vi "Restarts Sandbox New.vi"() -> ()   [LabVIEW 2013]
uses:
  Type Defs/CAN Mode.ctl
  Type Defs/Controller Names.ctl
  Type Defs/Controller List.ctl
  <vilib>/FPGAPlugInAG/sbRIO-9626/niLvFpga_Open_sbRIO-9626.vi
  <vilib>/rvi/interface/common/dynamic/niFpgaDynamicAddResources.vi
  <vilib>/rvi/interface/common/niFpgaWaitOnOcc.vi
  <vilib>/Utility/error.llb/Error Cluster From Error Code.vi
  <vilib>/rvi/errors/niLvFpgaAdjustHostInterfaceError.vi
  <vilib>/FPGAPlugInAG/Dynamic/niLvFpga_Reset_Dynamic.vi
  <vilib>/FPGAPlugInAG/Dynamic/niLvFpga_Run_Dynamic.vi
  <vilib>/rvi/interface/nirviOpenFPGA/nirviOpenFPGA.xnode
  FPGA/bitfiles/New Restarts Sandbox.lvbitx
  <vilib>/rvi/interface/nirviMethod/nirviMethod.xnode
  <vilib>/rvi/interface/nirviReadWriteControl/nirviReadWriteControl.xnode
  NiFpgaLv.dll
  <vilib>/rvi/interface/Simulation/niFpgaSimulationCallBeginRW.vi
  <vilib>/NI_Real-Time Target Support.lvlib
  <vilib>/FPGAPlugInAG/Dynamic/niLvFpga_ReadFifo_Dynamic.vi
  <vilib>/rvi/errors/niLvFpgaMergeErrorWithErrorCode.vi
  <vilib>/FPGAPlugInAG/Dynamic/niLvFpga_ConfigureFifo_Dynamic.vi
panel:
  out "RT rstrts":dbl
  out "FPGA rstrts":dbl
  in  "Tab Control":enum32{"Page 1", "Page 2"}(tab)
  out "Current Graph":dbl[](graph)
  out "Pressure Graph":dbl[](graph)
  out "Restarts Graph":dbl[](graph)
  out "graph":dbl[][](graph)
  out "Snapshot Graph":dbl[][](graph)
  in  "HighLimit":dbl=13614.0 format="%#_17g"
  in  "LowLimit":dbl=13208.0 format="%#_17g"
  in  "Trigger Span":i32=5
  out "Tracker":u32
  in  "Update Graphs":bool
  in  "Snapshot":bool
  out "Data Array":dbl[][](array[numeric])
  out "Pressure":dbl
  out "DetPres Starts":u32
  out "Current":fxp<+/-,28,17>
  out "Commanded Starts":i16
  in  "Position":i32=1
  in  "Seconds per Step":dbl=1.5 min=0.25 max=500.0 step=0.25
  out "Case":string
  out "Current Step":i32
  in  "Reset Restarts":bool
  in  "Profile":dbl[][](array[numeric])=[[1.25, 0.0, 0.0], [1.25, 650.0, 700.0]]
  in  "Run profile?":bool
  out "CFR 2":u64 format="%.0x"
  in  "Pressure":dbl min=0.0 max=800.0 step=1.0 format="%#_13g"
  out "CPU Usage:":dbl=7.74131899555212 format="%.1f"
  in  "CAN CMD":dbl min=0.0 max=800.0 step=1.0
  # "13238"
  # "13413"
  # "cmd"
  # "pres"
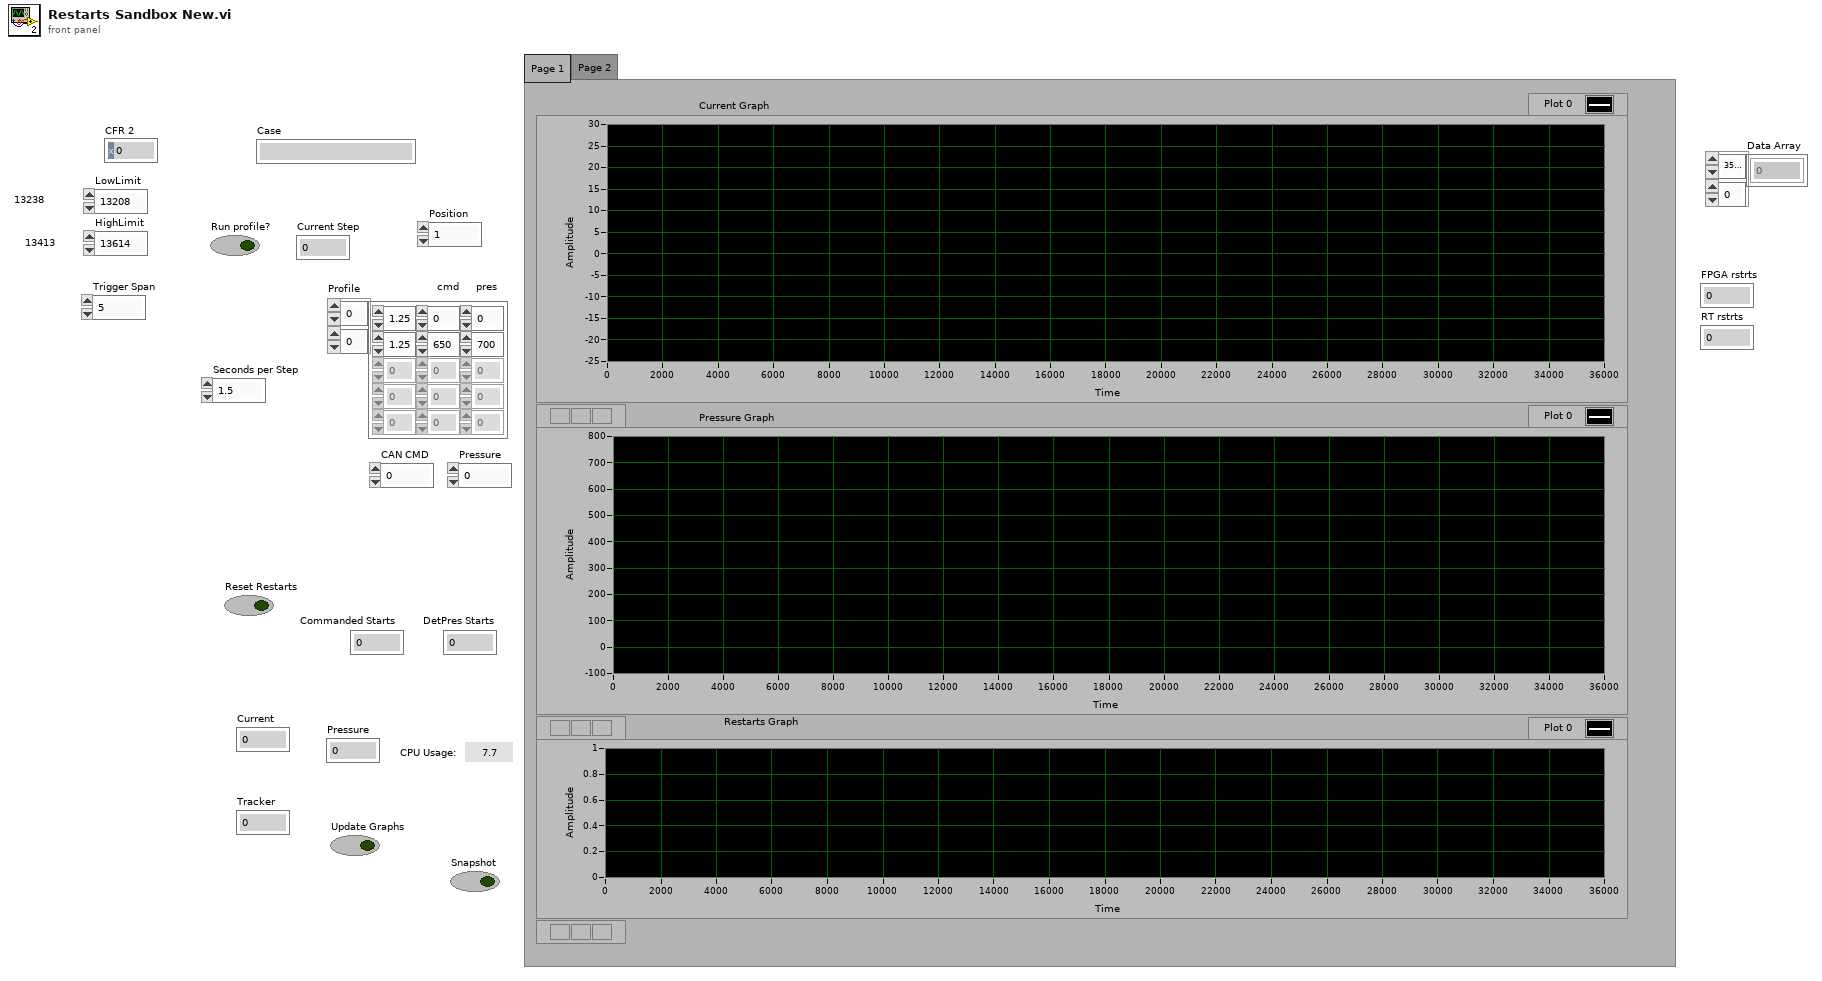
[diagram p1: front panel]
types:
  T1 = typedef "CAN Mode.ctl" = enum16{"Init", "Read", "Write", "Close"}
  T2 = cluster{"Container":dbl[], "Tracker":u32, "Curr1":dbl[], "Curr2":dbl[], "Curr3":dbl[], "Curr4":dbl[], "Curr5":dbl[], "Curr6":dbl[], "Pres1":dbl[], "Pres2":dbl[], "Pres3":dbl[], "Pres4":dbl[], "Pres5":dbl[], "Pres6":dbl[], "Restart1":dbl[], "Restart2":dbl[], "Restart3":dbl[], "Restart4":dbl[], "Restart5":dbl[], "Restart6":dbl[]}
  T3 = typedef "Controller Names.ctl" = enum16{"Kuhnke", "Conti", "Helbako", "TI PWM", "PSA", "Hella Gas", "Hella Diesel", "8 Comm", "10 Comm", "8 Comm Hella", "10 Comm Hella", "8 Comm Omron", "10 Comm Omron", "8 Comm Nissan", "10 Comm Nissan"}
  T4 = cluster{"Divide Value":u8, "Transfer Length (bits)":u8, "CS Asserted Polarity":bool, "Clock Polarity (CPOL)":bool, "Clock Phase (CPHA)":bool, "Lengthen MISO Setup":bool, "Direction Change Bit":u8, "MOSI Starts as Output":bool, "Tristatable MOSI":bool}
  T5 = typedef "Controller List.ctl" = cluster{"Controller Name":T3, "CommSeg":i32, "PWM?":bool, "Frequency":i32, "Low Command":dbl, "High Command":dbl, "Stop Command":dbl, "Command Step":dbl, "Solenoid Stop?":bool, "Controller?":bool}[]
  T6 = cluster{"Controller Name":T3, "CommSeg":i32, "PWM?":bool, "Frequency":i32, "Low Command":dbl, "High Command":dbl, "Stop Command":dbl, "Command Step":dbl, "Solenoid Stop?":bool, "Controller?":bool}
  T7 = typedef "NI_Real-Time Target Support.lvlib/RT CPU Load.ctl" = cluster{"Total (%)":dbl, "Time Critical (%)":dbl, "Timed Structures (%)":dbl, "High (%)":dbl, "Above Normal (%)":dbl, "Normal (%)":dbl, "Background (%)":dbl, "Idle (%)":dbl, "ISR (%)":dbl}
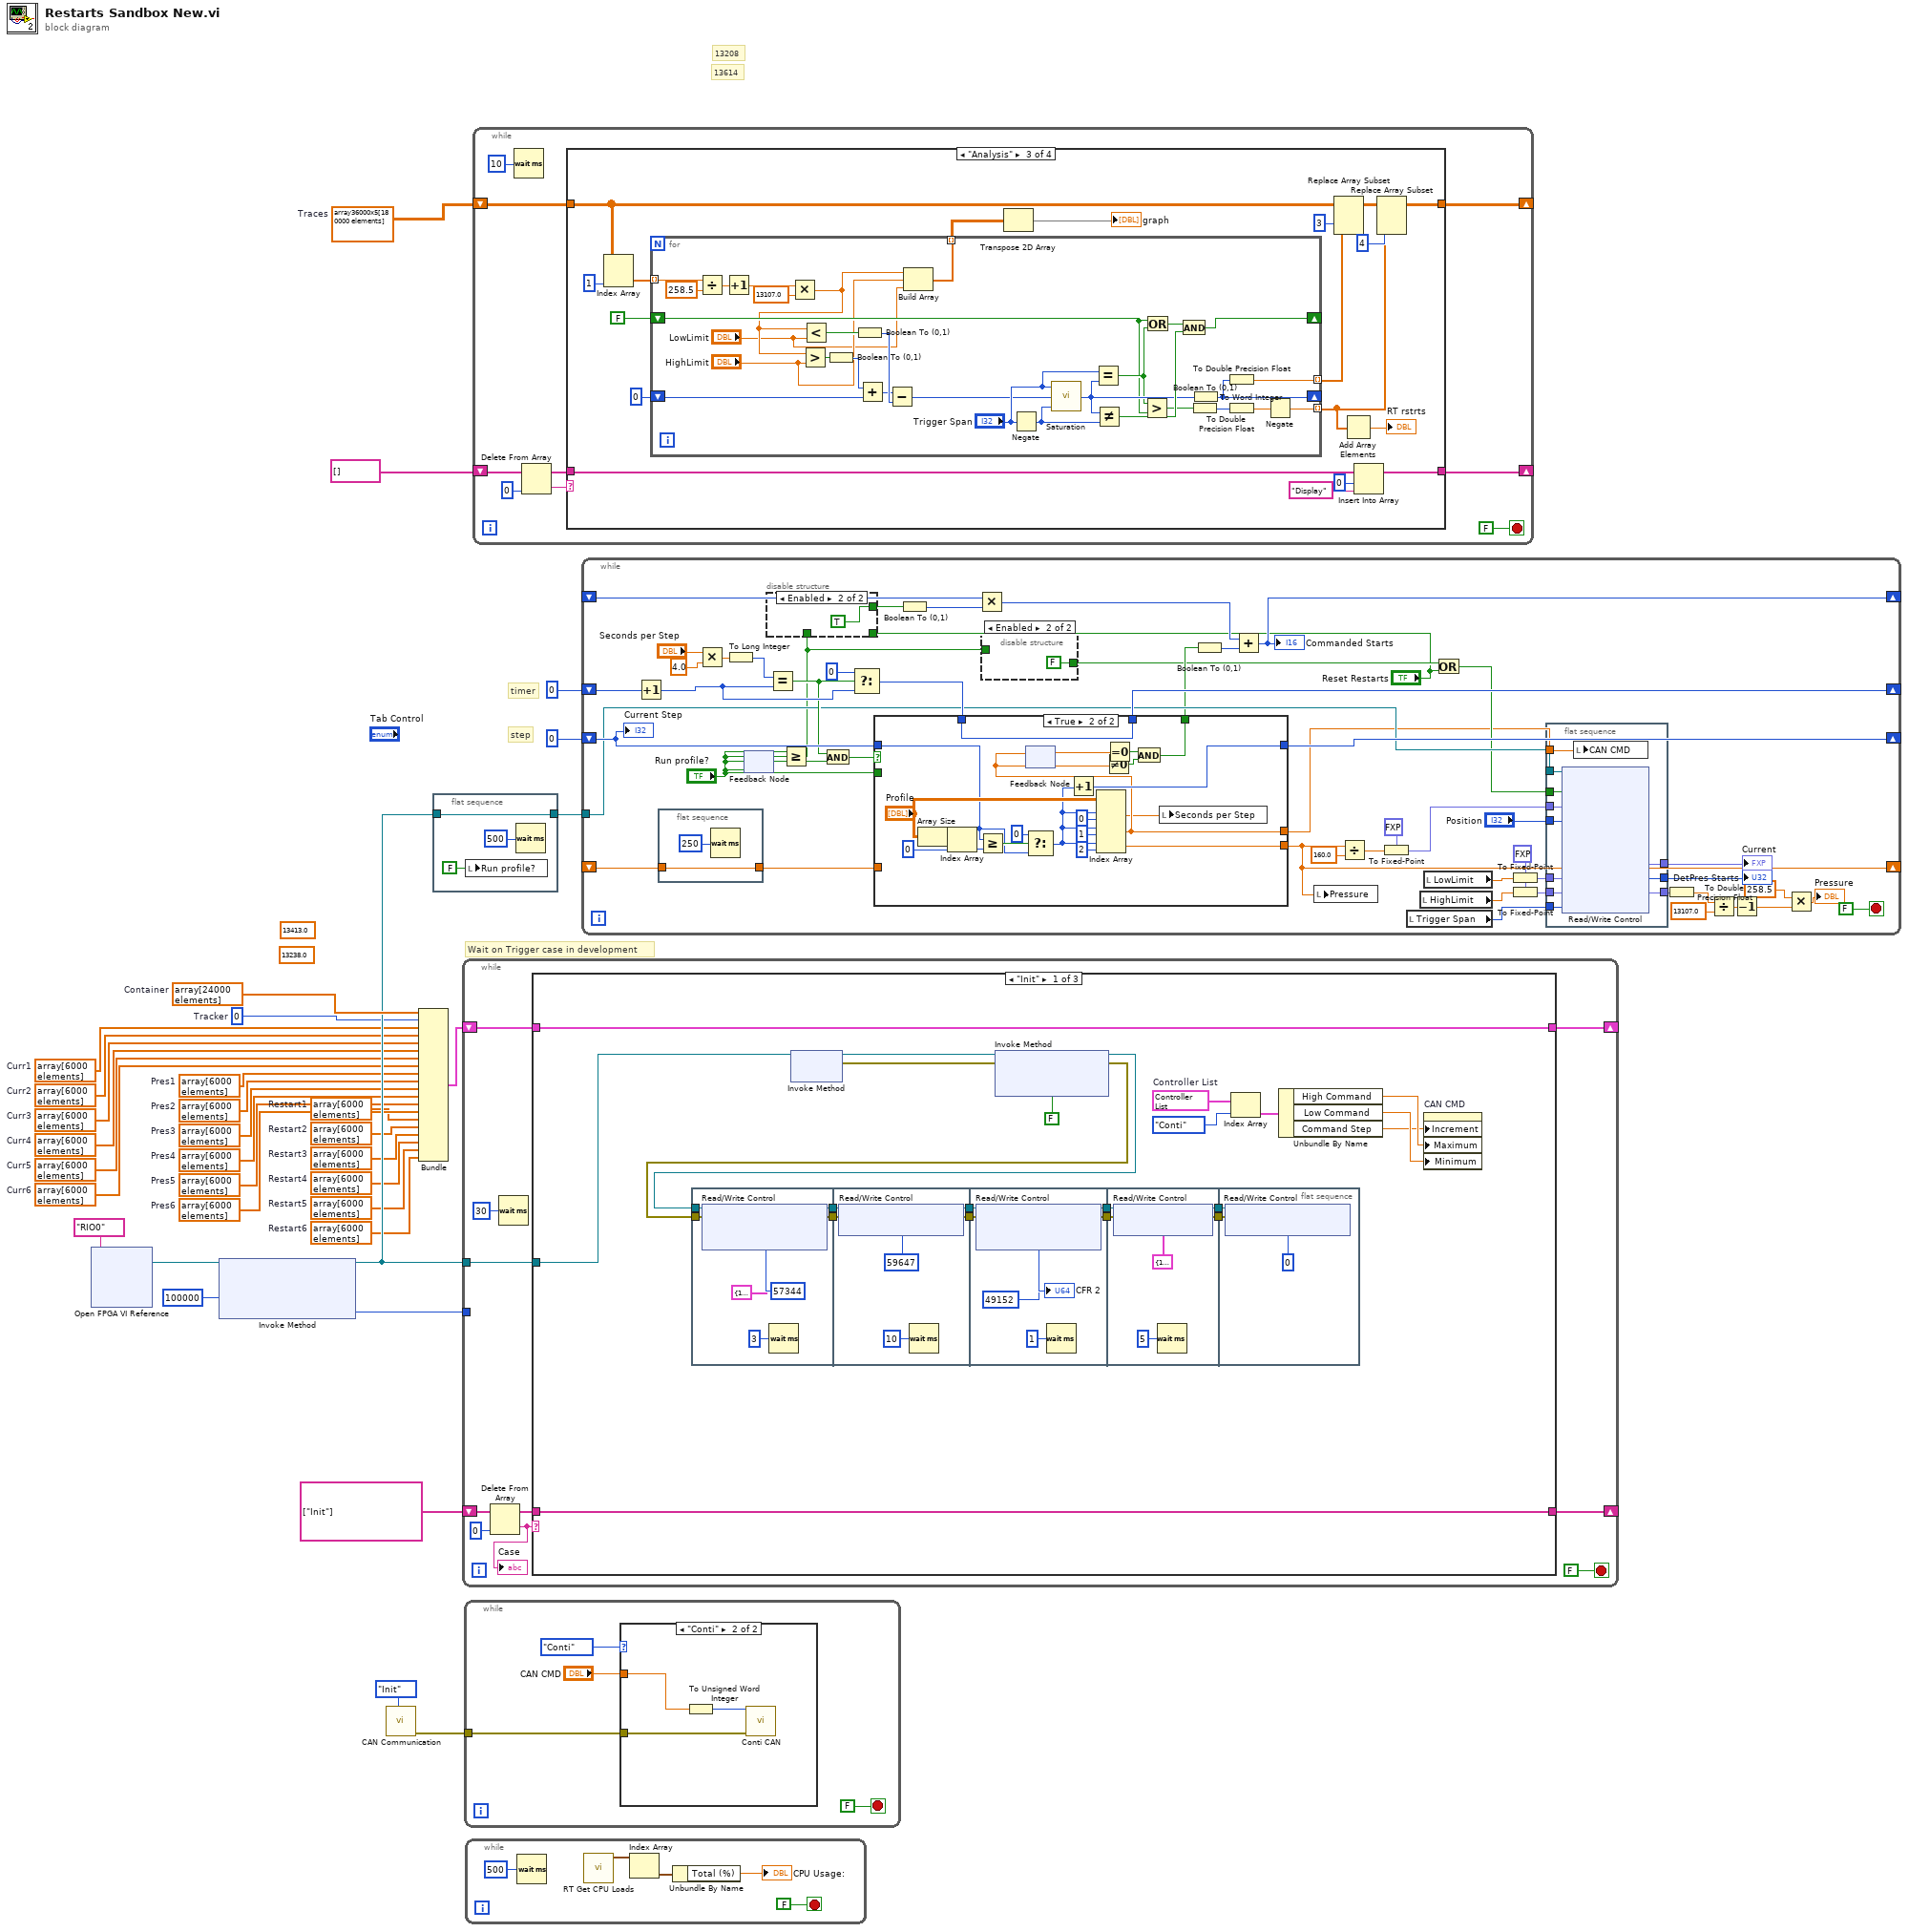
[diagram p0: block diagram]
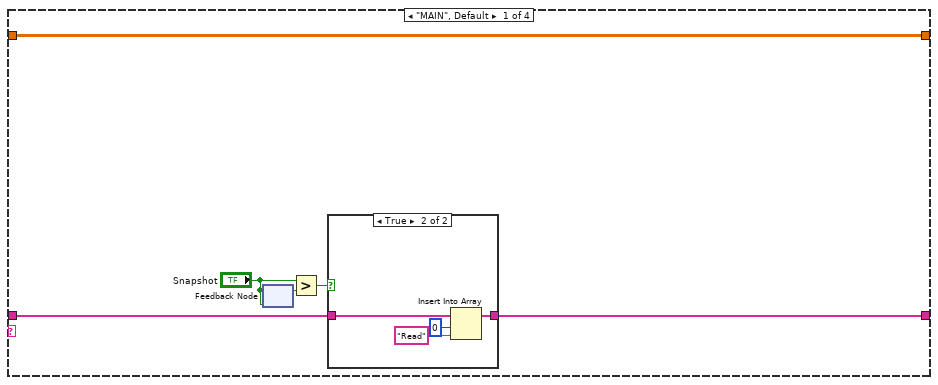
[diagram p2: hidden frame]
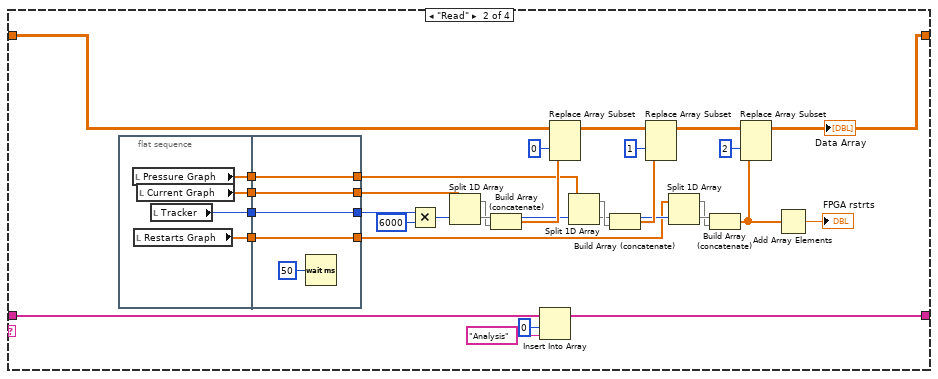
[diagram p4: hidden frame]
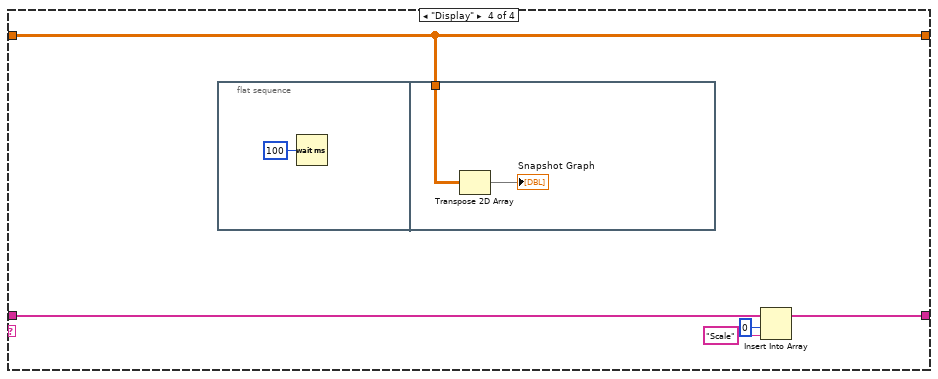
[diagram p5: hidden frame]
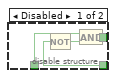
[diagram p6: hidden frame]
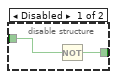
[diagram p7: hidden frame]
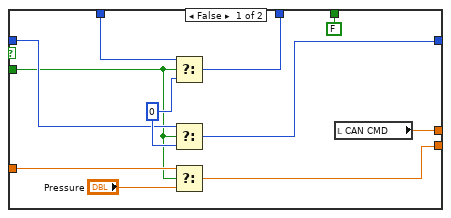
[diagram p8: hidden frame]
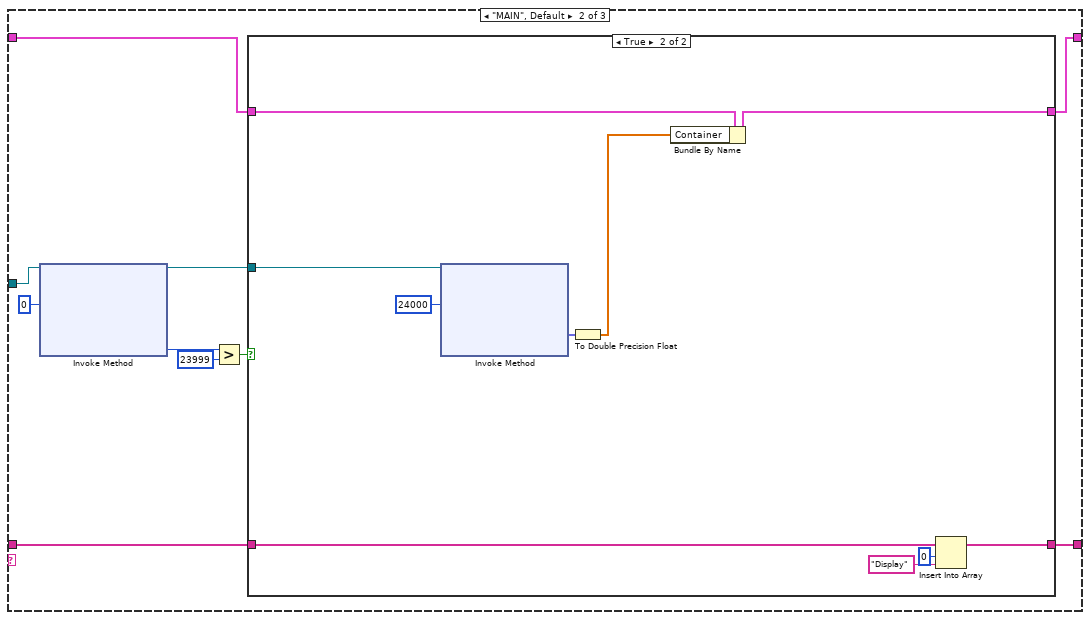
[diagram p9: hidden frame]
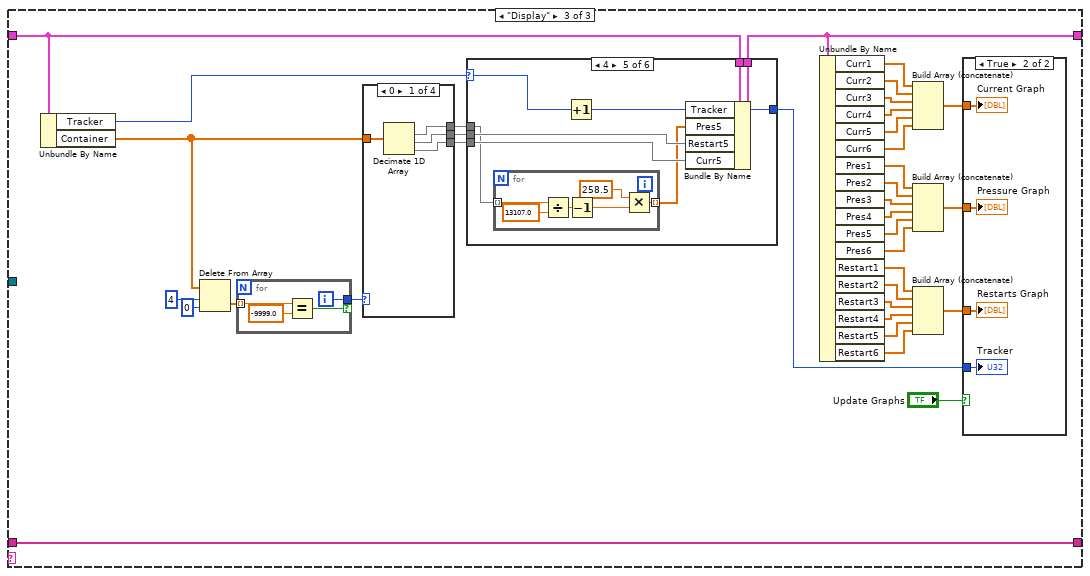
[diagram p11: hidden frame]
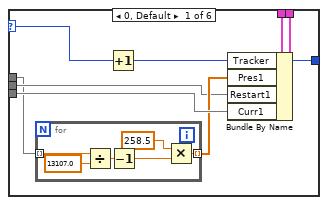
[diagram p13: hidden frame]
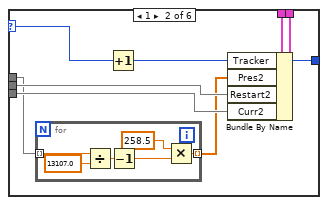
[diagram p14: hidden frame]
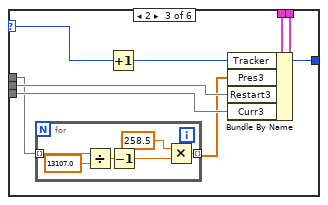
[diagram p15: hidden frame]
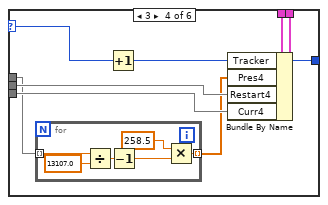
[diagram p16: hidden frame]
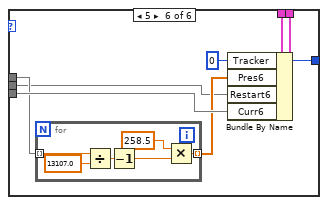
[diagram p17: hidden frame]
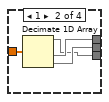
[diagram p18: hidden frame]
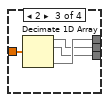
[diagram p19: hidden frame]
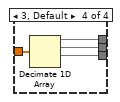
[diagram p20: hidden frame]
diagram:
  w2 = dbl[][] array36000x5[180000 elements]  # Traces
  w3 = dbl[] array[6000 elements]  # Restart6
  w4 = dbl[] array[6000 elements]  # Restart5
  w5 = dbl[] array[6000 elements]  # Restart4
  w6 = dbl[] array[6000 elements]  # Restart3
  w7 = dbl[] array[6000 elements]  # Restart2
  w8 = dbl[] array[6000 elements]  # Restart1
  w9 = dbl[] array[6000 elements]  # Pres6
  w10 = dbl[] array[6000 elements]  # Pres5
  w11 = dbl[] array[6000 elements]  # Pres4
  w12 = dbl[] array[6000 elements]  # Pres3
  w13 = dbl[] array[6000 elements]  # Pres2
  w14 = dbl[] array[6000 elements]  # Pres1
  w15 = dbl[] array[6000 elements]  # Curr6
  w16 = dbl[] array[6000 elements]  # Curr5
  w17 = dbl[] array[6000 elements]  # Curr4
  w18 = dbl[] array[6000 elements]  # Curr3
  w19 = dbl[] array[6000 elements]  # Curr2
  w20 = dbl[] array[6000 elements]  # Curr1
  (unwired) 13413.0 ("element")
  (unwired) 13238.0 ("element")
  w22 = u32 0  # Tracker
  w26 = dbl[] array[24000 elements]  # Container
  # "13614"
  # "13208"
  # "timer"
  # "step"
  # "Wait on Trigger case in development"
  n1 = xnode "Open FPGA VI Reference"("resource name"=tag "RIO0") -> ("FPGA VI Reference Out"=w28:refnum<k20>)  [unwired: 1 in, 1 out]
  n2 = xnode "Invoke Method"("FPGA VI Reference In"=w28, "Requested Depth"=u32 100000) -> ("FPGA VI Reference Out"=w25:refnum<k20>, "Actual Depth"=w27:u32)  [unwired: 1 in, 1 out]
  n3 = call "CAN Communication.vi"("CAN Mode"=CAN_Mode."Init") -> ("Error OUT"=w32:errorcluster)  [unwired: 10 in]
  n4 = Bundle("Container"=w26, "Tracker"=w22, "Curr1"=w20, "Curr2"=w19, "Curr3"=w18, "Curr4"=w17, "Curr5"=w16, "Curr6"=w15, "Pres1"=w14, "Pres2"=w13, "Pres3"=w12, "Pres4"=w11, "Pres5"=w10, "Pres6"=w9, "Restart1"=w8, "Restart2"=w7, "Restart3"=w6, "Restart4"=w5, "Restart5"=w4, "Restart6"=w3) -> (w30:T2)  [unwired: 1 in]
  n5 = flat-sequence {
    tunnel: w25 -> [w37]
    tunnel: [w37] -> w21
    frame #0 {
      n6 = local write "Run profile?"(FALSE ("Run profile?")) -> ()
      n7 = Wait (ms)(milliseconds to wait=u32 500) -> ()  [unwired: 1 out]
    }
  }
  n8 = while {
    shift-right: [w44] -> _
    shift-left: string[] ["Init"] -> [w47]
    shift-right: [w41] -> _
    shift-left: w30 -> [w42]
    tunnel: w25 -> [w40]
    tunnel: w27 -> [_]
    stop <- FALSE stop-if-true
    n9 = Delete From Array(array=w47, index=0) -> (deleted portion=w38:string, array with subset deleted=w45:string[])  [unwired: 1 in]
    "Case" <- w38
    n10 = Wait (ms)(milliseconds to wait=u32 30) -> ()  [unwired: 1 out]
    n11 = case shown="\"Init\"" w38 {
      tunnel: w45 -> [w69 w104 w154]
      tunnel: [w69 w103 w154] -> w44
      tunnel: w42 -> [w68 w101 w149]
      tunnel: [w68 w100 w121] -> w41
      tunnel: w40 -> [w67 w108 _]
      frame "Init" {
        w49 = T5 [{"Controller Name"=enum."Kuhnke", "CommSeg"=2, "PWM?"=TRUE, "Frequency"=100, "Low Command"=10.0, "High Command"=100.0, "Stop Command"=10.0, "Command Step"=0.1, "Solenoid Stop?"=FALSE, "Controller?"=FALSE}, {"Controller Name"=enum."Conti", "CommSeg"=2, "PWM?"=FALSE, "Frequency"=100, "Low Command"=0.0, "High Command"=800.0, "Stop Command"=0.0, "Command Step"=1.0, "Solenoid Stop?"=FALSE, "Controller?"=FALSE}, {"Controller Name"=enum."Helbako", "CommSeg"=2, "PWM?"=FALSE, "Frequency"=100, "Low Command"=0.0, "High Command"=100.0, "Stop Command"=0.0, "Command Step"=0.1, "Solenoid Stop?"=FALSE, "Controller?"=FALSE}, {"Controller Name"=enum."TI PWM", "CommSeg"=2, "PWM?"=TRUE, "Frequency"=100, "Low Command"=0.0, "High Command"=100.0, "Stop Command"=0.0, "Command Step"=0.1, "Solenoid Stop?"=FALSE, "Controller?"=FALSE}, {"Controller Name"=enum."PSA", "CommSeg"=2, "PWM?"=TRUE, "Frequency"=100, "Low Command"=5.0, "High Command"=95.0, "Stop Command"=5.0, "Command Step"=0.1, "Solenoid Stop?"=FALSE, "Controller?"=FALSE}, {"Controller Name"=enum."Hella Gas", "CommSeg"=2, "PWM?"=FALSE, "Frequency"=100, "Low Command"=0.0, "High Command"=800.0, "Stop Command"=0.0, "Command Step"=1.0, "Solenoid Stop?"=TRUE, "Controller?"=FALSE}, {"Controller Name"=enum."Hella Diesel", "CommSeg"=2, "PWM?"=FALSE, "Frequency"=100, "Low Command"=370.0, "High Command"=461.0, "Stop Command"=370.0, "Command Step"=1.0, "Solenoid Stop?"=TRUE, "Controller?"=FALSE}, {"Controller Name"=enum."8 Comm", "CommSeg"=8, "PWM?"=FALSE, "Frequency"=100, "Low Command"=0.0, "High Command"=1.0, "Stop Command"=0.0, "Command Step"=1.0, "Solenoid Stop?"=FALSE, "Controller?"=FALSE}, {"Controller Name"=enum."10 Comm", "CommSeg"=10, "PWM?"=FALSE, "Frequency"=100, "Low Command"=0.0, "High Command"=1.0, "Stop Command"=0.0, "Command Step"=1.0, "Solenoid Stop?"=FALSE, "Controller?"=FALSE}, {"Controller Name"=enum."8 Comm Hella", "CommSeg"=8, "PWM?"=TRUE, "Frequency"=150, "Low Command"=0.0, "High Command"=50.0, "Stop Command"=80.0, "Command Step"=0.1, "Solenoid Stop?"=FALSE, "Controller?"=FALSE}, {"Controller Name"=enum."10 Comm Hella", "CommSeg"=10, "PWM?"=TRUE, "Frequency"=150, "Low Command"=0.0, "High Command"=50.0, "Stop Command"=80.0, "Command Step"=0.1, "Solenoid Stop?"=FALSE, "Controller?"=FALSE}, {"Controller Name"=enum."8 Comm Omron", "CommSeg"=8, "PWM?"=TRUE, "Frequency"=150, "Low Command"=5.0, "High Command"=50.0, "Stop Command"=75.0, "Command Step"=0.1, "Solenoid Stop?"=FALSE, "Controller?"=FALSE}, {"Controller Name"=enum."10 Comm Omron", "CommSeg"=10, "PWM?"=TRUE, "Frequency"=150, "Low Command"=5.0, "High Command"=50.0, "Stop Command"=75.0, "Command Step"=0.1, "Solenoid Stop?"=FALSE, "Controller?"=FALSE}, {"Controller Name"=enum."8 Comm Nissan", "CommSeg"=8, "PWM?"=TRUE, "Frequency"=10, "Low Command"=50.0, "High Command"=90.0, "Stop Command"=50.0, "Command Step"=0.1, "Solenoid Stop?"=TRUE, "Controller?"=FALSE}, {"Controller Name"=enum."10 Comm Nissan", "CommSeg"=10, "PWM?"=TRUE, "Frequency"=10, "Low Command"=50.0, "High Command"=90.0, "Stop Command"=50.0, "Command Step"=0.1, "Solenoid Stop?"=TRUE, "Controller?"=FALSE}]  # Controller List
        n12 = flat-sequence {
          tunnel: w53 -> [w75]
          tunnel: w52 -> [w73]
          tunnel: [w76] -> w61
          tunnel: [w74] -> w60
          tunnel: w61 -> [w81]
          tunnel: w60 -> [w80]
          tunnel: [w79] -> w59
          tunnel: [w78] -> w58
          tunnel: w59 -> [w88]
          tunnel: w58 -> [w87]
          tunnel: [w86] -> w57
          tunnel: [w85] -> w56
          tunnel: w57 -> [w94]
          tunnel: w56 -> [w93]
          tunnel: [w91] -> w55
          tunnel: [w90] -> w54
          tunnel: w55 -> [w97]
          tunnel: w54 -> [w96]
          frame #0 {
            n13 = xnode "Read/Write Control"("FPGA VI Reference In"=w75, "error in"=w73, "AI16-23 Settings"=T4 {"Divide Value"=1, "Transfer Length (bits)"=16, "CS Asserted Polarity"=FALSE, "Clock Polarity (CPOL)"=TRUE, "Clock Phase (CPHA)"=FALSE, "Lengthen MISO Setup"=FALSE, "Direction Change Bit"=0, "MOSI Starts as Output"=FALSE, "Tristatable MOSI"=FALSE} ("Master Settings"), "AI16-23 Data to Write"=u64 57344 ("data to write")) -> ("FPGA VI Reference Out"=w76:refnum<k20>, "error out"=w74:errorcluster)
            n14 = Wait (ms)(milliseconds to wait=u32 3) -> ()  [unwired: 1 out]
          }
          frame #1 {
            n15 = xnode "Read/Write Control"("FPGA VI Reference In"=w81, "error in"=w80, "AI16-23 Data to Write"=u64 59647 ("data to write")) -> ("FPGA VI Reference Out"=w79:refnum<k20>, "error out"=w78:errorcluster)
            n16 = Wait (ms)(milliseconds to wait=u32 10) -> ()  [unwired: 1 out]
          }
          frame #2 {
            n17 = xnode "Read/Write Control"("FPGA VI Reference In"=w88, "error in"=w87, "AI16-23 Data to Write"=u64 49152 ("data to write")) -> ("FPGA VI Reference Out"=w86:refnum<k20>, "error out"=w85:errorcluster, "Read Data"=→"CFR 2":u64)
            n18 = Wait (ms)(milliseconds to wait=u32 1) -> ()  [unwired: 1 out]
          }
          frame #3 {
            n19 = xnode "Read/Write Control"("FPGA VI Reference In"=w94, "error in"=w93, "AI16-23 Settings"=T4 {"Divide Value"=1, "Transfer Length (bits)"=19, "CS Asserted Polarity"=FALSE, "Clock Polarity (CPOL)"=TRUE, "Clock Phase (CPHA)"=FALSE, "Lengthen MISO Setup"=FALSE, "Direction Change Bit"=0, "MOSI Starts as Output"=FALSE, "Tristatable MOSI"=FALSE} ("Master Settings")) -> ("FPGA VI Reference Out"=w91:refnum<k20>, "error out"=w90:errorcluster)
            n20 = Wait (ms)(milliseconds to wait=u32 5) -> ()  [unwired: 1 out]
          }
          frame #4 {
            n21 = xnode "Read/Write Control"("FPGA VI Reference In"=w97, "error in"=w96, "AI16-23 Data to Write"=u64 0) -> ()  [unwired: 2 out]
          }
        }
        n22 = xnode "Invoke Method"("FPGA VI Reference In"=w67) -> ("FPGA VI Reference Out"=w51:refnum<k20>, "error out"=w50:errorcluster)  [unwired: 1 in]
        n23 = xnode "Invoke Method"("FPGA VI Reference In"=w51, "error in"=w50, "Wait Until Done (F)"=FALSE) -> ("FPGA VI Reference Out"=w53:refnum<k20>, "error out"=w52:errorcluster)
        n24 = Index Array(array=w49, index=Controller_Names."Conti" ("Controller Type:")) -> (element=w63:T6)
        n25 = Unbundle By Name(w63) -> ("High Command"=w66:dbl, "Low Command"=w65:dbl, "Command Step"=w64:dbl)
        n26 = property on="CAN CMD" class="DigNum (strict)"("Increment"=w64, "Maximum"=w66, "Minimum"=w65) -> ()  [unwired: 2 in, 2 out]
      }
      frame "MAIN", Default {
        n27 = xnode "Invoke Method"("FPGA VI Reference In"=w108, "Number of Elements"=u32 0) -> ("FPGA VI Reference Out"=w99:refnum<k20>, "Elements Remaining"=w106:u32)  [unwired: 2 in, 2 out]
        n28 = Greater?(x=w106, y=u32 23999) -> (0:w102:bool)
        n29 = case shown="True" w102 {
          tunnel: w104 -> [w110 w118]
          tunnel: [w110 w117] -> w103
          tunnel: w101 -> [w109 w120]
          tunnel: [w109 w119] -> w100
          tunnel: w99 -> [_ w115]
          frame False {
          }
          frame True {
            n30 = xnode "Invoke Method"("FPGA VI Reference In"=w115, "Number of Elements"=u32 24000) -> ("Data"=w116:fxp<+/-,28,17>[])  [unwired: 2 in, 3 out]
            n31 = To Double Precision Float(number=w116) -> (double precision float=w113:dbl[])
            n32 = Bundle By Name(cluster=w120, "Container"=w113) -> (w119:T2)
            n33 = Insert Into Array(array=w118, index=0, new element="Display" ("new element/subarray")) -> (w117:string[])
          }
        }
      }
      frame "Display" {
        n34 = Unbundle By Name(w149) -> ("Tracker"=w124:u32, "Container"=w150:dbl[])
        n35 = Delete From Array(array=w150, length=4, index=0) -> (deleted portion=w152:dbl[])  [unwired: 1 out]
        n36 = for {
          tunnel: w152 -> [w261] mode=indexing
          tunnel: [w262] -> w151 if=w259
          i -> [w262]
          n37 = Equal?(x=w261, y=-9999.0) -> (x = y?=w259:bool)
        }
        n38 = case shown="0" w151 {
          tunnel: w150 -> [w246 w250 w254 w258]
          tunnel: [w245 w249 w253 w257] -> w127
          tunnel: [w244 w248 w252 w256] -> w126
          tunnel: [w243 w247 w251 w255] -> w125
          frame 0 {
            n39 = Decimate 1D Array(w246) -> (w245:dbl[], w244:dbl[], w243:dbl[])  [unwired: 1 out]
          }
          frame 1 {
            n40 = Decimate 1D Array(w250) -> (w247:dbl[], w249:dbl[], w248:dbl[])  [unwired: 1 out]
          }
          frame 2 {
            n41 = Decimate 1D Array(w254) -> (w252:dbl[], w251:dbl[], w253:dbl[])  [unwired: 1 out]
          }
          frame 3, Default {
            n42 = Decimate 1D Array(w258) -> (w257:dbl[], w256:dbl[], w255:dbl[])  [unwired: 1 out]
          }
        }
        n43 = case shown="4" w124 {
          selector: w124 -> [w164 w178 w192 w206 w220 _]
          tunnel: w127 -> [w161 w176 w189 w203 w217 w233]
          tunnel: w126 -> [w162 w177 w191 w205 w219 w231]
          tunnel: w125 -> [w166 w180 w194 w208 w222 w235]
          tunnel: w149 -> [w167 w181 w195 w209 w223 w236]
          tunnel: [w165 w179 w193 w207 w221 w234] -> w121
          tunnel: [w160 w174 w188 w202 w216 w230] -> w122
          frame 0, Default {
            n44 = for {
              tunnel: w161 -> [w169] mode=indexing
              tunnel: [w168] -> w163 mode=indexing
              n45 = Divide(x=w169, y=13107.0) -> (x/y=w171:dbl)
              n46 = Decrement(x=w171) -> (x-1=w172:dbl)
              n47 = Multiply(x=258.5, y=w172) -> (x*y=w168:dbl)
            }
            n48 = Increment(x=w164) -> (x+1=w160:u32)
            n49 = Bundle By Name(cluster=w167, "Tracker"=w160, "Pres1"=w163, "Restart1"=w162, "Curr1"=w166) -> (w165:T2)
          }
          frame 1 {
            n50 = for {
              tunnel: w176 -> [w183] mode=indexing
              tunnel: [w182] -> w175 mode=indexing
              n51 = Divide(x=w183, y=13107.0) -> (x/y=w185:dbl)
              n52 = Decrement(x=w185) -> (x-1=w186:dbl)
              n53 = Multiply(x=258.5, y=w186) -> (x*y=w182:dbl)
            }
            n54 = Increment(x=w178) -> (x+1=w174:u32)
            n55 = Bundle By Name(cluster=w181, "Tracker"=w174, "Pres2"=w175, "Restart2"=w177, "Curr2"=w180) -> (w179:T2)
          }
          frame 2 {
            n56 = for {
              tunnel: w189 -> [w197] mode=indexing
              tunnel: [w196] -> w190 mode=indexing
              n57 = Divide(x=w197, y=13107.0) -> (x/y=w199:dbl)
              n58 = Decrement(x=w199) -> (x-1=w200:dbl)
              n59 = Multiply(x=258.5, y=w200) -> (x*y=w196:dbl)
            }
            n60 = Increment(x=w192) -> (x+1=w188:u32)
            n61 = Bundle By Name(cluster=w195, "Tracker"=w188, "Pres3"=w190, "Restart3"=w191, "Curr3"=w194) -> (w193:T2)
          }
          frame 3 {
            n62 = for {
              tunnel: w203 -> [w211] mode=indexing
              tunnel: [w210] -> w204 mode=indexing
              n63 = Divide(x=w211, y=13107.0) -> (x/y=w213:dbl)
              n64 = Decrement(x=w213) -> (x-1=w214:dbl)
              n65 = Multiply(x=258.5, y=w214) -> (x*y=w210:dbl)
            }
            n66 = Increment(x=w206) -> (x+1=w202:u32)
            n67 = Bundle By Name(cluster=w209, "Tracker"=w202, "Pres4"=w204, "Restart4"=w205, "Curr4"=w208) -> (w207:T2)
          }
          frame 4 {
            n68 = for {
              tunnel: w217 -> [w225] mode=indexing
              tunnel: [w224] -> w218 mode=indexing
              n69 = Divide(x=w225, y=13107.0) -> (x/y=w227:dbl)
              n70 = Decrement(x=w227) -> (x-1=w228:dbl)
              n71 = Multiply(x=258.5, y=w228) -> (x*y=w224:dbl)
            }
            n72 = Increment(x=w220) -> (x+1=w216:u32)
            n73 = Bundle By Name(cluster=w223, "Tracker"=w216, "Pres5"=w218, "Restart5"=w219, "Curr5"=w222) -> (w221:T2)
          }
          frame 5 {
            w230 = u32 0 ("Tracker")
            n74 = for {
              tunnel: w233 -> [w238] mode=indexing
              tunnel: [w237] -> w232 mode=indexing
              n75 = Divide(x=w238, y=13107.0) -> (x/y=w240:dbl)
              n76 = Decrement(x=w240) -> (x-1=w241:dbl)
              n77 = Multiply(x=258.5, y=w241) -> (x*y=w237:dbl)
            }
            n78 = Bundle By Name(cluster=w236, "Tracker"=w230, "Pres6"=w232, "Restart6"=w231, "Curr6"=w235) -> (w234:T2)
          }
        }
        n79 = Unbundle By Name(w121) -> ("Curr1"=w141:dbl[], "Curr2"=w142:dbl[], "Curr3"=w146:dbl[], "Curr4"=w145:dbl[], "Curr5"=w140:dbl[], "Curr6"=w139:dbl[], "Pres1"=w138:dbl[], "Pres2"=w137:dbl[], "Pres3"=w143:dbl[], "Pres4"=w144:dbl[], "Pres5"=w136:dbl[], "Pres6"=w135:dbl[], "Restart1"=w134:dbl[], "Restart2"=w133:dbl[], "Restart3"=w147:dbl[], "Restart4"=w148:dbl[], "Restart5"=w132:dbl[], "Restart6"=w131:dbl[])
        n80 = Build Array (concatenate)(w141, w142, w146, w145, w140, w139) -> (w128:dbl[])
        n81 = Build Array (concatenate)(w138, w137, w143, w144, w136, w135) -> (w130:dbl[])
        n82 = Build Array (concatenate)(w134, w133, w147, w148, w132, w131) -> (w129:dbl[])
        n83 = case shown="True" "Update Graphs" {
          tunnel: w130 -> [_ w159]
          tunnel: w129 -> [_ w158]
          tunnel: w128 -> [_ w157]
          tunnel: w122 -> [_ w156]
          frame False {
          }
          frame True {
            "Restarts Graph" <- w158
            "Current Graph" <- w157
            "Pressure Graph" <- w159
            "Tracker" <- w156
          }
        }
      }
    }
  }
  n84 = while {
    tunnel: w32 -> [w265]
    stop <- FALSE stop-if-true
    n85 = case shown="\"Conti\"" Controller_Names."Conti" ("Controller Type:") {
      tunnel: w265 -> [_ w270]
      tunnel: "CAN CMD" -> [_ w269]
      frame "Kuhnke", Default {
        n86 = Wait (ms)(milliseconds to wait=u32 500) -> ()  [unwired: 1 out]
      }
      frame "Conti" {
        n87 = To Unsigned Word Integer(number=w269) -> (unsigned 16bit integer=w268:u16)
        n88 = call "Conti CAN.vi"("Error IN"=w270, "CMD"=w268) -> ()  [unwired: 9 in, 1 out]
      }
    }
  }
  n89 = while {
    stop <- FALSE stop-if-true
    n90 = Wait (ms)(milliseconds to wait=u32 500) -> ()  [unwired: 1 out]
    n91 = call <vilib>:"RT Get CPU Loads.vi"() -> ("CPU loads"=w272:T7[])  [unwired: 10 in, 1 out]
    n92 = Index Array(array=w272) -> (element=w273:T7)  [unwired: 1 in]
    n93 = Unbundle By Name(w273) -> ("Total (%)"=→"CPU Usage:":dbl)
  }
  n94 = while {
    shift-right: [w277] -> _
    shift-left: w2 -> [w278]
    shift-right: [w276] -> _
    shift-left: string[] [] -> [w282]
    stop <- FALSE stop-if-true
    n95 = Wait (ms)(milliseconds to wait=u32 10) -> ()  [unwired: 1 out]
    n96 = Delete From Array(array=w282, index=0) -> (deleted portion=w279:string, array with subset deleted=w280:string[])  [unwired: 1 in]
    n97 = case shown="\"Analysis\"" w279 {
      tunnel: w280 -> [w286 w303 w341 w385]
      tunnel: w278 -> [w290 w326 w349 w388]
      tunnel: [w290 w325 w347 w388] -> w277
      tunnel: [w285 w302 w340 w384] -> w276
      frame "MAIN", Default {
        n98 = feedback-in #1("Snapshot") -> ()
        n99 = feedback #1("Snapshot") -> (w289:bool)
        n100 = Greater?(x="Snapshot", y=w289) -> (0:w287:bool)
        n101 = case shown="True" w287 {
          tunnel: w286 -> [w291 w293]
          tunnel: [w291 w292] -> w285
          frame False {
          }
          frame True {
            n102 = Insert Into Array(array=w293, index=0, new element="Read" ("new element/subarray")) -> (w292:string[])
          }
        }
      }
      frame "Read" {
        n103 = flat-sequence {
          tunnel: [w330] -> w301
          tunnel: [w329] -> w300
          tunnel: [w328] -> w299
          tunnel: [w327] -> w298
          tunnel: [w332] -> w306
          tunnel: [w333] -> w307
          tunnel: [w334] -> w308
          tunnel: [w335] -> w309
          tunnel: w301 -> [w335]
          tunnel: w300 -> [w334]
          tunnel: w299 -> [w333]
          tunnel: w298 -> [w332]
          frame #0 {
            n104 = local read "Pressure Graph"() -> (w328:dbl[])
            n105 = local read "Restarts Graph"() -> (w327:dbl[])
            n106 = local read "Current Graph"() -> (w329:dbl[])
            n107 = local read "Tracker"() -> (w330:u32)
          }
          frame #1 {
            n108 = Wait (ms)(milliseconds to wait=u32 50) -> ()  [unwired: 1 out]
          }
        }
        n109 = Multiply(x=w309, y=u32 6000) -> (x*y=w310:u32)
        n110 = Split 1D Array(array=w308, index=w310) -> (first subarray=w317:dbl[], second subarray=w318:dbl[])
        n111 = Build Array (concatenate)(w318, w317) -> (w311:dbl[])
        n112 = Insert Into Array(array=w303, index=0, new element="Analysis" ("new element/subarray")) -> (w302:string[])
        n113 = Replace Array Subset(array=w326, new element=w311, index (col)=0 ("disabled index (col)")) -> (w321:dbl[][])  [unwired: 1 in]
        n114 = Split 1D Array(array=w307, index=w310) -> (first subarray=w316:dbl[], second subarray=w315:dbl[])
        n115 = Build Array (concatenate)(w315, w316) -> (w312:dbl[])
        n116 = Replace Array Subset(array=w321, new element=w312, index (col)=1) -> (w320:dbl[][])  [unwired: 1 in]
        n117 = Split 1D Array(array=w306, index=w310) -> (first subarray=w313:dbl[], second subarray=w314:dbl[])
        n118 = Build Array (concatenate)(w314, w313) -> (w297:dbl[])
        n119 = Replace Array Subset(array=w320, new element=w297, index (col)=2) -> (w325:dbl[][])  [unwired: 1 in]
        "Data Array" <- w325
        n120 = Add Array Elements(numeric array=w297) -> (sum=→"FPGA rstrts":dbl)
      }
      frame "Analysis" {
        n121 = Index Array(array=w349, index (col)=1 ("disabled index (col)")) -> (element=w352:dbl[])  [unwired: 1 in]
        n122 = for {
          tunnel: w352 -> [w383] mode=indexing
          shift-right: [w371] -> _
          shift-left: FALSE -> [w360]
          shift-right: [w362] -> _
          shift-left: i16 0 -> [w365]
          tunnel: [w358] -> w337 mode=indexing
          tunnel: [w361] -> w344 mode=indexing
          tunnel: [w356] -> w339 mode=indexing
          n123 = Divide(x=w383, y=258.5 ("x")) -> (x/y=w381:dbl)
          n124 = Increment(x=w381) -> (x+1=w380:dbl)
          n125 = Multiply(x=w380, y=13107.0) -> (x*y=w357:dbl)
          n126 = Greater?(x=w357, y="HighLimit") -> (0:w374:bool)
          n127 = Less?(x=w357, y="LowLimit") -> (x < y?=w373:bool)
          n128 = Boolean To (0,1)(Boolean=w374) -> (0, 1=w377:i16)
          n129 = Boolean To (0,1)(Boolean=w373) -> (0, 1=w378:i16)
          n130 = Add(x=w377, y=w365) -> (x+y=w372:i16)
          n131 = Subtract(x=w372, y=w378) -> (x-y=w369:i16)
          n132 = Build Array(w357, "HighLimit", "LowLimit") -> (w356:dbl[])
          n133 = Negate(x="Trigger Span") -> (-x=w368:i32)
          n134 = call "Saturation"("upper limit"="Trigger Span", "input"=w369, "lower limit"=w368) -> ("output"=w367:i32)  [unwired: 6 in]
          n135 = Equal?(x="Trigger Span", y=w367) -> (x = y?=w366:bool)
          n136 = Not Equal?(x=w367, y=w368) -> (x != y?=w376:bool)
          n137 = Greater?(x=w366, y=w360) -> (0:w364:bool)
          n138 = Or(x=w360, y=w366) -> (x .or. y?=w375:bool)
          n139 = And(x=w375, y=w376) -> (x .and. y?=w371:bool)
          n140 = Boolean To (0,1)(Boolean=w364) -> (0, 1=w363:i16)
          n141 = To Word Integer(number=w367) -> (16bit integer=w362:i16)
          n142 = To Double Precision Float(number=w362) -> (double precision float=w361:dbl)
          n143 = To Double Precision Float(number=w363) -> (double precision float=w359:dbl)
          n144 = Negate(x=w359) -> (-x=w358:dbl)
        }
        n145 = Transpose 2D Array(2D array=w339) -> (transposed array=→"graph":dbl[][])
        n146 = Replace Array Subset(array=w349, new element=w344, index (col)=3 ("disabled index (col)")) -> (w348:dbl[][])  [unwired: 1 in]
        n147 = Add Array Elements(numeric array=w337) -> (sum=→"RT rstrts":dbl)
        n148 = Insert Into Array(array=w341, index=0, new element="Display" ("new element/subarray")) -> (w340:string[])
        n149 = Replace Array Subset(array=w348, new element=w337, index (col)=4 ("disabled index (col)")) -> (w347:dbl[][])  [unwired: 1 in]
      }
      frame "Display" {
        n150 = flat-sequence {
          tunnel: w388 -> [w391]
          frame #0 {
            n151 = Wait (ms)(milliseconds to wait=u32 100) -> ()  [unwired: 1 out]
          }
          frame #1 {
            n152 = Transpose 2D Array(2D array=w391) -> (transposed array=→"Snapshot Graph":dbl[][])
          }
        }
        n153 = Insert Into Array(array=w385, index=0, new element="Scale" ("new element/subarray")) -> (w384:string[])
      }
    }
  }
  n154 = while {
    tunnel: w21 -> [w425]
    shift-right: [w437] -> _
    shift-left: 0 ("disabled index (col)") -> [w438]
    shift-right: [w432] -> _
    shift-left: 0 ("disabled index (col)") -> [w436]
    shift-right: [w410] -> _
    shift-left: _ -> [w430]
    shift-right: [w421] -> _
    shift-left: _ -> [w419]
    stop <- FALSE stop-if-true
    w395 = fxp<+/-,28,17> 0.0 ("LowLimit")
    n155 = Increment(x=w436) -> (x+1=w431:i32)
    n156 = flat-sequence {
      tunnel: w430 -> [w464]
      tunnel: [w464] -> w429
      frame #0 {
        n157 = Wait (ms)(milliseconds to wait=u32 250) -> ()  [unwired: 1 out]
      }
    }
    n158 = Multiply(x="Seconds per Step", y=4.0) -> (x*y=w415:dbl)
    n159 = To Long Integer(number=w415) -> (32bit integer=w414:i32)
    n160 = feedback #2("Run profile?") -> (w416:bool)
    n161 = feedback-in #2("Run profile?") -> ()
    n162 = Equal?(x=w414, y=w431) -> (x = y?=w428:bool)
    n163 = Greater Or Equal?(x="Run profile?", y=w416) -> (x >= y?=w409:bool)
    n164 = disable-structure shown="Enabled" {
      disable-tunnel: w409 -> [w447 _]
      disable-tunnel: [w446 TRUE] -> w408
      disable-tunnel: "Reset Restarts" -> [w445 _]
      frame Disabled {
        n165 = Not(x=w445) -> (.not. x?=w444:bool)
        n166 = And(x=w447, y=w444) -> (x .and. y?=w446:bool)
      }
      frame Enabled {
      }
    }
    n167 = And(x=w428, y="Run profile?") -> (x .and. y?=w435:bool)
    n168 = Select(t=0, s=w428, f=w431) -> (s? t:f=w433:i32)
    n169 = case shown="True" w435 {
      tunnel: [w471 w493] -> w410
      tunnel: w438 -> [w469 w486]
      tunnel: [w467 w484] -> w437
      tunnel: w433 -> [w475 w485]
      tunnel: [w474 w485] -> w432
      tunnel: "Run profile?" -> [w468 _]
      tunnel: w429 -> [w473 _]
      tunnel: [FALSE w483] -> w423
      tunnel: [w465 w479] -> w411
      frame False {
        w470 = 0 ("disabled index (col)")
        n170 = Select(t=w475, s=w468, f=w470) -> (s? t:f=w474:i32)
        n171 = Select(t=w469, s=w468, f=w470) -> (s? t:f=w467:i32)
        n172 = Select(t=w473, s=w468, f="Pressure") -> (s? t:f=w471:dbl)
        n173 = local read "CAN CMD"() -> (w465:dbl)
      }
      frame True {
        n174 = Array Size(array="Profile") -> (size(s)=w491:i32[])
        n175 = Index Array(array=w491, index=0 ("disabled index (col)")) -> (element=w489:i32)
        n176 = Greater Or Equal?(x=w486, y=w489) -> (x >= y?=w488:bool)
        n177 = Select(t=0, s=w488, f=w486) -> (s? t:f=w478:i32)
        n178 = Increment(x=w478) -> (x+1=w484:i32)
        n179 = Index Array(array="Profile", index (row) #1=w478, index (col) #1=0 ("disabled index (col)"), index (row) #2=w478, index (col) #2=1 ("disabled index (col)"), index (row) #3=w478, index (col) #3=2 ("disabled index (col)")) -> (element #1=w476:dbl, element #2=w479:dbl, element #3=w493:dbl)
        n180 = feedback-in #3(w479) -> ()
        n181 = feedback #3(w479) -> (w480:dbl)
        n182 = Not Equal To 0?(x=w479) -> (x != 0?=w481:bool)
        n183 = Equal To 0?(x=w480) -> (x = 0?=w482:bool)
        n184 = And(x=w482, y=w481) -> (x .and. y?=w483:bool)
        n185 = local write "Seconds per Step"(w476) -> ()
      }
    }
    n186 = Boolean To (0,1)(Boolean=w408) -> (0, 1=w420:i16)
    n187 = Multiply(x=w419, y=w420) -> (x*y=w418:i16)
    n188 = disable-structure shown="Enabled" {
      disable-tunnel: [w450 FALSE] -> w413
      disable-tunnel: w409 -> [w449 _]
      frame Disabled {
        n189 = Not(x=w449) -> (.not. x?=w450:bool)
      }
      frame Enabled {
      }
    }
    n190 = Boolean To (0,1)(Boolean=w423) -> (0, 1=w422:i16)
    n191 = Add(x=w418, y=w422) -> (x+y=w421:i16)
    "Commanded Starts" <- w421
    n192 = local write "Pressure"(w410) -> ()
    n193 = Divide(x=w410, y=160.0) -> (x/y=w440:dbl)
    n194 = To Fixed-Point(fixed-point type=fxp<+/-,20,5> 0.0 ("AO0"), number=w440) -> (fixed-point=w439:fxp<+/-,20,5>)
    n195 = local read "Trigger Span"() -> (w394:i32)
    n196 = local read "HighLimit"() -> (w393:dbl)
    n197 = local read "LowLimit"() -> (w392:dbl)
    n198 = Or(x=w413, y="Reset Restarts") -> (x .or. y?=w412:bool)
    n199 = To Fixed-Point(fixed-point type=w395, number=w392) -> (fixed-point=w397:fxp<+/-,28,17>)
    n200 = To Fixed-Point(fixed-point type=w395, number=w393) -> (fixed-point=w396:fxp<+/-,28,17>)
    n201 = flat-sequence {
      tunnel: w439 -> [w462]
      tunnel: w425 -> [w461]
      tunnel: "Position" -> [w460]
      tunnel: w412 -> [w459]
      tunnel: w411 -> [w458]
      tunnel: [w457] -> w406
      tunnel: [w456] -> w405
      tunnel: [w455] -> w404
      tunnel: w397 -> [w454]
      tunnel: w396 -> [w453]
      tunnel: w394 -> [w452]
      frame #0 {
        n202 = xnode "Read/Write Control"("FPGA VI Reference In"=w461, "Reset Restarts"=w459, "AO0"=w462, "Position"=w460, "LowLimit"=w454, "HighLimit"=w453, "Trigger Span"=w452) -> ("Current"=w457:fxp<+/-,28,17>, "DetPres Starts"=w456:u32, "Pressure"=w455:fxp<+/-,28,17>)  [unwired: 1 in, 2 out]
        n203 = local write "CAN CMD"(w458) -> ()
      }
    }
    n204 = To Double Precision Float(number=w404) -> (double precision float=w398:dbl)
    n205 = Divide(x=w398, y=13107.0) -> (x/y=w401:dbl)
    n206 = Decrement(x=w401) -> (x-1=w402:dbl)
    n207 = Multiply(x=258.5, y=w402) -> (x*y=→"Pressure":dbl)
    "Current Step" <- w438
    "Current" <- w406
    "DetPres Starts" <- w405
  }
